vi "ConvertCToF.vi"(1 "deg C":dbl) -> (0 "deg F":dbl)   [LabVIEW 2025]
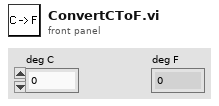
[diagram p1: front panel]
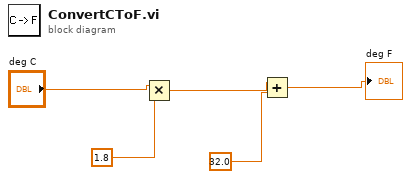
[diagram p0: block diagram]
diagram:
  n1 = Multiply(x="deg C", y=1.8) -> (x*y=w4:dbl)
  n2 = Add(x=w4, y=32.0) -> (x+y=→"deg F":dbl)
